vi "averaging_data.vi"(6 "Offset":dbl, 9 "Input":dbl[](array[numeric])) -> (0 "Offset Average":dbl, 2 "Input Out":dbl[](array[numeric]), 3 "Average":dbl, 5 "Input Offset":dbl[](array[numeric]))   [LabVIEW 2017]
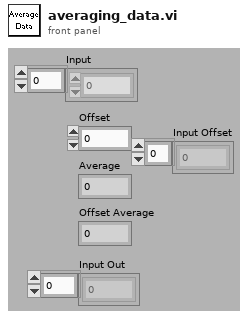
[diagram p1: front panel]
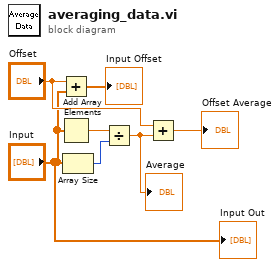
[diagram p0: block diagram]
diagram:
  n1 = Add(x="Offset", y="Input") -> (x+y=→"Input Offset":dbl[])
  n2 = Add Array Elements(numeric array="Input") -> (sum=w4:dbl)
  n3 = Array Size(array="Input") -> (size(s)=w3:i32)
  n4 = Divide(x=w4, y=w3) -> (x/y=w2:dbl)
  "Average" <- w2
  n5 = Add(x="Offset", y=w2) -> (x+y=→"Offset Average":dbl)
  "Input Out" <- "Input"
